vi "To Waveform.vi"(8 "error in (no error)":errorcluster, 11 "Test Double Data in":refnum<class "Test Double Data.lvclass">) -> (0 "error out":errorcluster, 1 "Success?":bool, 3 "Waveform Array":waveform(dbl)[](array[waveform]))   [LabVIEW 2020, in "Test.lvlib" / "Test Double Data.lvclass"]
doc: "Interpret 'Data' as a Waveform Array. If impossible 'Success?' is set to FALSE"
uses:
  Test Double Data.lvclass
  Test Double Data.lvclass/Test Double Data.ctl
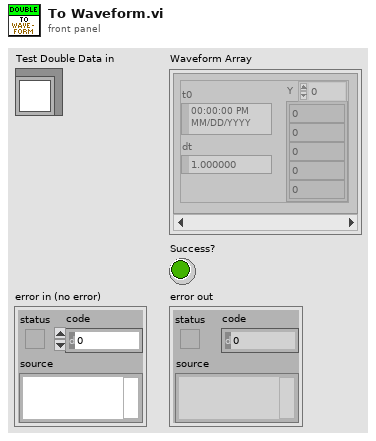
[diagram p1: front panel]
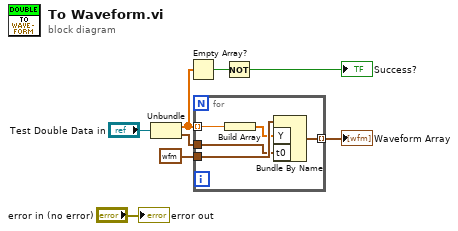
[diagram p0: block diagram]
diagram:
  n1 = Unbundle("Test Double Data in") -> (w4:dbl[], w6:timestamp)
  n2 = Empty Array?(array=w4) -> (empty?=w3:bool)
  n3 = for {
    tunnel: waveform(dbl) {"t0"=timestamp(0 s since 1904-01-01), "dt"=1.0, "Y"=[]} ("Waveform Array") -> [w13]
    tunnel: w4 -> [w12] mode=indexing
    tunnel: w6 -> [w10]
    tunnel: [w9] -> w5 mode=indexing
    n4 = Build Array(w12) -> (w11:dbl[])
    n5 = Bundle By Name(cluster=w13, "Y"=w11, "t0"=w10) -> (w9:waveform(dbl))
  }
  "Waveform Array" <- w5
  n6 = Not(x=w3) -> (.not. x?=→"Success?":bool)
  "error out" <- "error in (no error)"
